vi "get_component_type_name.vi"(8 "error in (no error)":errorcluster, 11 "GenericScanHead in":refnum<class "GenericScanHead.lvclass">) -> (0 "error out":errorcluster, 2 "component type":string, 3 "GenericScanHead out":refnum<class "GenericScanHead.lvclass">)   [LabVIEW 2010, in "GenericScanHead.lvclass"]
uses:
  GenericScanHead.lvclass
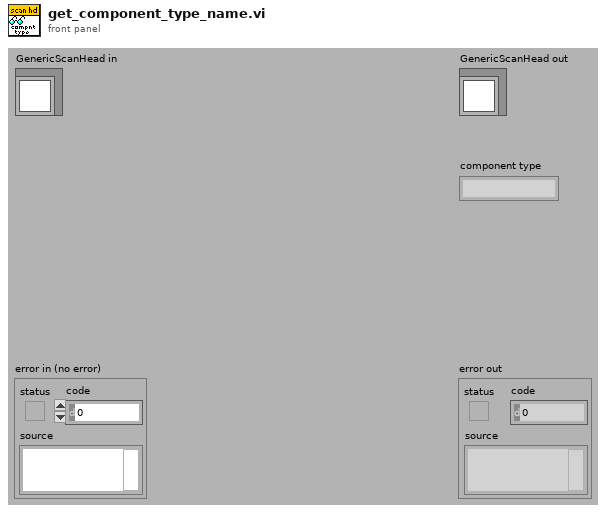
[diagram p1: front panel]
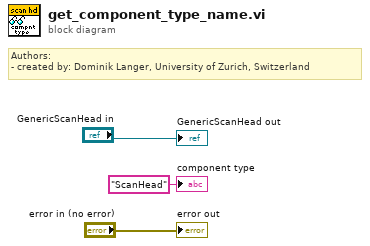
[diagram p0: block diagram]
diagram:
  # "Authors: \n- created by: Dominik Langer, University of Zurich, Switzerland"
  "error out" <- "error in (no error)"
  "GenericScanHead out" <- "GenericScanHead in"
  "component type" <- "ScanHead" ("component type")
